vi "KeysightVOLTCURR.vi"(8 "error in (no error)":errorcluster, 9 "CURR/VOLT (A/V)":dbl, 10 "CURR (1)/VOLT (0)":bool, 11 "VISA resource name":refnum<visa-resource-name>) -> (0 "error out":errorcluster, 3 "VISA resource name out":refnum<visa-resource-name>)   [LabVIEW 2017]
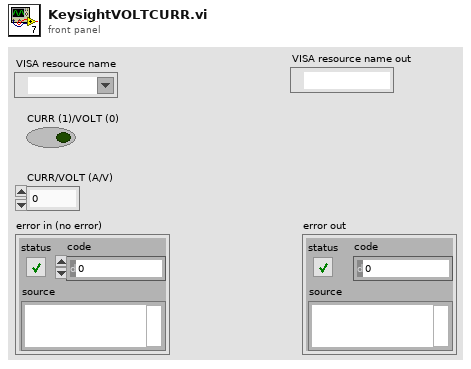
[diagram p1: front panel]
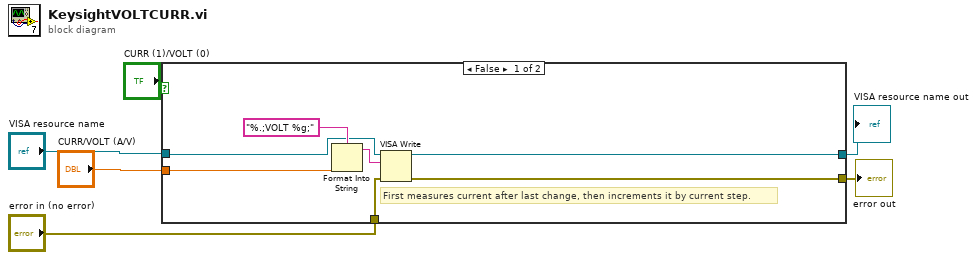
[diagram p0: block diagram]
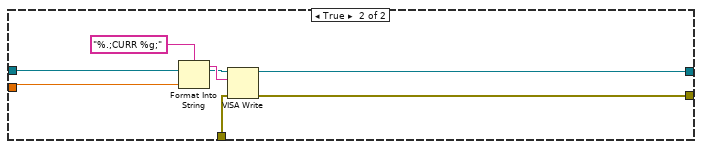
[diagram p2: hidden frame]
diagram:
  n1 = case shown="False" "CURR (1)/VOLT (0)" {
    tunnel: [w11 w18] -> w1
    tunnel: [w10 w17] -> w2
    tunnel: "CURR/VOLT (A/V)" -> [w9 w16]
    tunnel: "VISA resource name" -> [w8 w15]
    tunnel: "error in (no error)" -> [w7 w14]
    frame False {
      # "First measures current after last change, then increments it by current step."
      n2 = Format Into String(format string="%.;VOLT %g;", w9) -> (resulting string=w12:string)  [unwired: 2 in, 1 out]
      n3 = VISA Write(VISA resource name=w8, write buffer=w12, error in (no error)=w7) -> (VISA resource name out=w11:refnum<visa-resource-name>, error out=w10:errorcluster)  [unwired: 1 out]
    }
    frame True {
      n4 = Format Into String(format string="%.;CURR %g;", w16) -> (resulting string=w19:string)  [unwired: 2 in, 1 out]
      n5 = VISA Write(VISA resource name=w15, write buffer=w19, error in (no error)=w14) -> (VISA resource name out=w18:refnum<visa-resource-name>, error out=w17:errorcluster)  [unwired: 1 out]
    }
  }
  "error out" <- w2
  "VISA resource name out" <- w1
